vi "BRig_dataCurrent_idxDataTrial.vi"() -> (2 "output_idxDataTrial":i32)   [LabVIEW 2014]
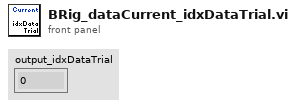
[diagram p1: front panel]
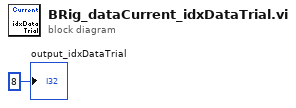
[diagram p0: block diagram]
diagram:
  "output_idxDataTrial" <- 8 ("output_iBlock")
